vi "NI VeriStand - Unlock Connection.vi"(8 "error in (no error)":errorcluster, 10 "Password":string, 11 "WorkspaceManager in":T1) -> (0 "error out":errorcluster, 3 "WorkspaceManager out":T1)   [LabVIEW 2020, in "NI_VS Workspace ExecutionAPI.lvlib"]
doc: "Unlocks the current VeriStand Gateway connection."
uses:
  <vilib>/NI VeriStand/Execution/Workspace/NI_VS Workspace ExecutionAPI.lvlib
  <vilib>/NI VeriStand/Execution/Workspace/WorkspaceAPI.ctl
  NationalInstruments.VeriStand.ClientAPI
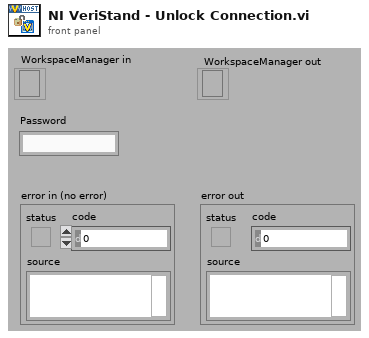
[diagram p1: front panel]
types:
  T1 = typedef "NI_VS Workspace ExecutionAPI.lvlib/WorkspaceAPI.ctl" = refnum<k24>
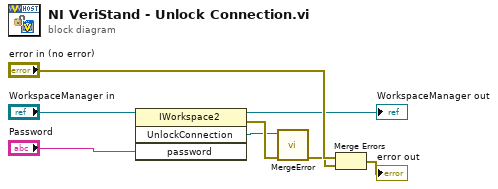
[diagram p0: block diagram]
diagram:
  n1 = invoke class="IWorkspace2" method="UnlockConnection"(reference="WorkspaceManager in", "password"="Password") -> (reference out=→"WorkspaceManager out":T1, error out=w8:errorcluster, "UnlockConnection"=w4:refnum<k24>)  [unwired: 2 in, 1 out]
  n2 = call <vilib>:"MergeError.vi"("error in (no error)"=w8, "Error"=w4) -> ("error out"=w2:errorcluster)  [unwired: 9 out]
  n3 = Merge Errors("error in (no error)", w2) -> (→"error out":errorcluster)
